vi "MoveServo_R3.vi"(6 "DIO Ref Out":T1, 8 "VISA resource name out":refnum<visa-resource-name>, 9 "GP - Low Byte":string=" ", 10 "GP - High Byte":string="\u0000", 11 "Servo ID":string="\u0001") -> (2 "Valid Checksum":bool=TRUE, 3 "Error":u64)   [LabVIEW 2015]
uses:
  <vilib>/myRIO/Instrument Drivers/Onboard IO/DIO/typedefs/DIO Reference.ctl
  <vilib>/myRIO/Common/Instrument Driver Framework/Utilities/typedefs/myRIO Generic Hardware Reference.ctl
  <vilib>/myRIO/Common/Instrument Driver Framework/Utilities/typedefs/Hardware Version Enum.ctl
  <vilib>/myRIO/Common/Instrument Driver Framework/Utilities/typedefs/myRIO v1.0 Reference.ctl
  <vilib>/myRIO/Common/Instrument Driver Framework/Utilities/typedefs/Generic FPGA Reference.ctl
  <vilib>/myRIO/Common/Instrument Driver Framework/myRIO v1.0/DIO/typedefs/DIO Channels List.ctl
  <vilib>/myRIO/Common/Instrument Driver Framework/myRIO v1.0/DIO/typedefs/DIO Channels Enum.ctl
  <vilib>/Utility/error.llb/Error Cluster From Error Code.vi
  <vilib>/myRIO/Common/Instrument Driver Framework/myRIO v1.0/DIO/vis/myRIO v1.0 Write DIO.vi
  <vilib>/myRIO/Instrument Drivers/Onboard IO/DIO/DIO.lvlib
panel:
  out "Checksum":string
  out "Tx Packet":string
  out "Calc Cksm":u8
  out "Received\nCksm":u8
  out "Received\nArray":u8[](array[numeric])
  in  "Transmit \nDelay (us)":i32=850
  in  "Return\nDelay (us)":i32=1000
  in  "RECEIVE (F)":bool[](array[boolean])=[FALSE]
  in  "TRANSMIT (T)":bool[](array[boolean])=[TRUE]
  out "Received String Array":string[](array[string])
  out "Received String":string
  # "SEND VALUES"
  # "RECEIVED VALUES"
  # "OUTPUT VALUES"
  # "INPUT"
  # "Config Parameters"
  # "Tx/Rx Delays"
  # "UART HW needs\n2-3ms to process signal\nkeeping at 2.5ms to be safe"
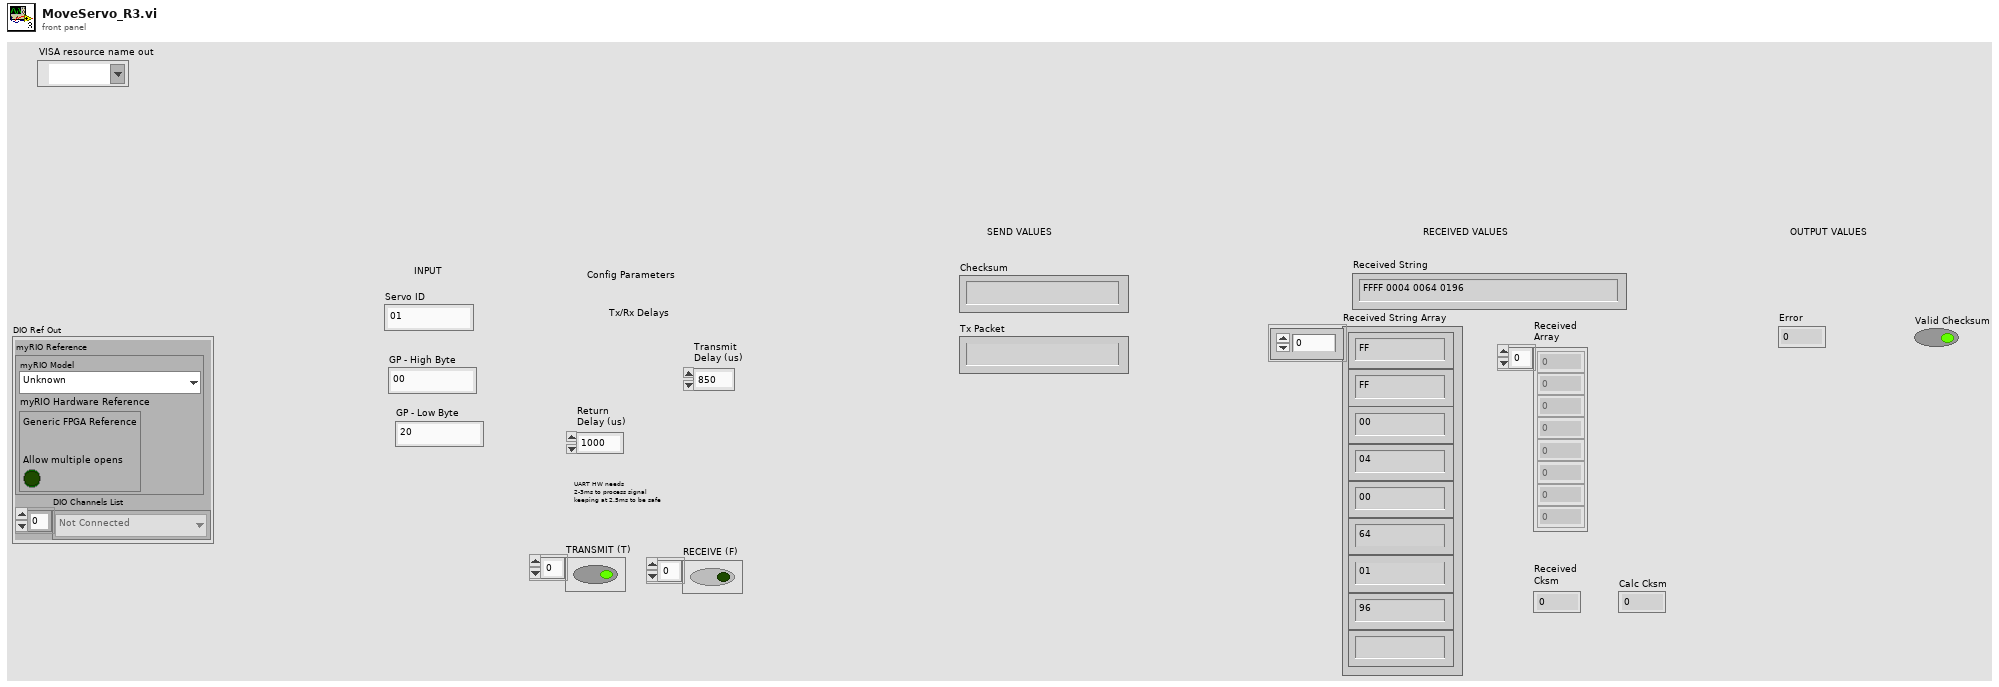
[diagram p1: front panel]
types:
  T1 = typedef "DIO.lvlib/DIO Reference.ctl" = cluster{"myRIO Reference":T2, "DIO Channels List":T6}
  T2 = typedef "myRIO Generic Hardware Reference.ctl" = cluster{"myRIO Model":T3, "myRIO Hardware Reference":T4}
  T3 = typedef "Hardware Version Enum.ctl" = enum16{"Unknown", "myRIO-1900", "myRIO-1950", "roboRIO"}
  T4 = typedef "myRIO v1.0 Reference.ctl" = cluster{"Generic FPGA Reference":T5, "Allow multiple opens":bool}
  T5 = typedef "Generic FPGA Reference.ctl" = refnum<k20>
  T6 = typedef "DIO Channels List.ctl" = T7[]
  T7 = typedef "DIO Channels Enum.ctl" = enum16{"Not Connected", "C/DIO0", "C/DIO1", "C/DIO2", "C/DIO3", "C/DIO4", "C/DIO5", "C/DIO6", "C/DIO7", "A/DIO0", "A/DIO1", "A/DIO2", "A/DIO3", "A/DIO4", "A/DIO5", "A/DIO6", "A/DIO7", "A/DIO8", "A/DIO9", "A/DIO10", "A/DIO11", "A/DIO12", "A/DIO13", "A/DIO14", "A/DIO15", "B/DIO0", "B/DIO1", "B/DIO2", "B/DIO3", "B/DIO4", "B/DIO5", "B/DIO6", "B/DIO7", "B/DIO8", "B/DIO9", "B/DIO10", "B/DIO11", "B/DIO12", "B/DIO13", "B/DIO14", "B/DIO15", "LED0", "LED1", "LED2", "LED3", "Button0", "DIO/DIO0", "DIO/DIO1", "DIO/DIO2", "DIO/DIO3", "DIO/DIO4", "DIO/DIO5", "DIO/DIO6", "DIO/DIO7", "DIO/DIO8", "DIO/DIO9", "SPI/CS0", "SPI/CS1", "SPI/CS2", "SPI/CS3", "LED RADIO (Green)", "LED RADIO (Red)", "LED COMM (Green)", "LED COMM (Red)", "LED MODE (Green)", "LED MODE (Red)"}
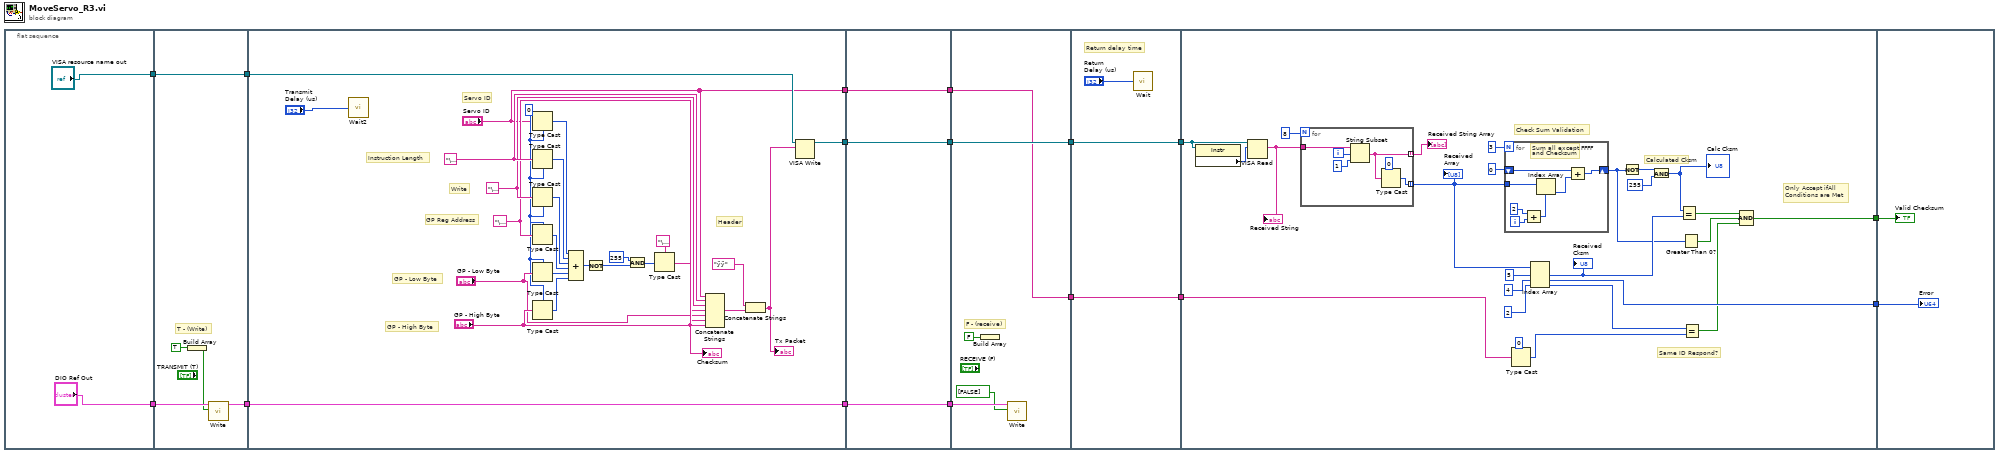
[diagram p0: block diagram]
diagram:
  n1 = flat-sequence {
    tunnel: ["VISA resource name out"] -> w16
    tunnel: ["DIO Ref Out"] -> w15
    tunnel: [w23] -> w14
    tunnel: [w20] -> w13
    tunnel: w16 -> [w20]
    tunnel: w15 -> [w21]
    tunnel: [w49] -> w12
    tunnel: [w47] -> w11
    tunnel: ["Servo ID"] -> w1
    tunnel: w13 -> [w48]
    tunnel: w14 -> [w49]
    tunnel: w12 -> [w52]
    tunnel: [w52] -> w10
    tunnel: w11 -> [w51]
    tunnel: [w51] -> w9
    tunnel: [w50] -> w2
    tunnel: w1 -> [w50]
    tunnel: w10 -> [w57]
    tunnel: w9 -> [w55]
    tunnel: [w55] -> w8
    tunnel: [w53] -> w3
    tunnel: w2 -> [w53]
    tunnel: w8 -> [w59]
    tunnel: [w59] -> w7
    tunnel: [w58] -> w4
    tunnel: w3 -> [w58]
    tunnel: w7 -> [w83]
    tunnel: [w61] -> w6
    tunnel: [w68] -> w5
    tunnel: w4 -> [w62]
    tunnel: w6 -> [w100]
    tunnel: w5 -> [w99]
    frame #0 {
    }
    frame #1 {
      # "T - (Write)"
      n2 = Build Array(TRUE) -> (w19:bool[])
      n3 = call <vilib>:"Write.vi"("Values"=w19, "DIO Ref In"=w21) -> ("DIO Ref Out"=w23:T1)  [unwired: 7 in, 1 out]
    }
    frame #2 {
      w29 = u8 0
      w34 = "\u001e"
      w35 = "\u0003"
      w36 = "\u0005"
      # "GP - High Byte"
      # "GP Reg Address"
      # "GP - Low Byte"
      # "Write"
      # "Instruction Length"
      # "Servo ID"
      # "Header"
      n4 = call "Wait2"("Count(uSec)"="Transmit \nDelay (us)") -> ()  [unwired: 1 out]
      n5 = Type Cast(type=w29, x="Servo ID") -> (*(type *) &x=w37:u8)
      n6 = Type Cast(type=w29, x=w36) -> (*(type *) &x=w38:u8)
      n7 = Type Cast(type=w29, x=w35) -> (*(type *) &x=w28:u8)
      n8 = Type Cast(type=w29, x=w34) -> (*(type *) &x=w39:u8)
      n9 = Type Cast(type=w29, x="GP - Low Byte") -> (*(type *) &x=w40:u8)
      n10 = Type Cast(type=w29, x="GP - High Byte") -> (*(type *) &x=w27:u8)
      n11 = Compound Arithmetic op=ADD(w37, w38, w28, w39, w40, w27) -> (w41:u8)
      n12 = Not(x=w41) -> (.not. x?=w43:u8)
      n13 = And(x=u8 255, y=w43) -> (x .and. y?=w45:u8)
      n14 = Type Cast(type="\u0000", x=w45) -> (*(type *) &x=w46:string)
      "Checksum" <- w46
      n15 = Concatenate Strings("Servo ID", w36, w35, w34, "GP - Low Byte", "GP - High Byte", w46) -> (w31:string)
      n16 = Concatenate Strings("ÿÿ", w31) -> (w26:string)
      "Tx Packet" <- w26
      n17 = VISA Write(VISA resource name=w48, write buffer=w26) -> (VISA resource name out=w47:refnum<visa-resource-name>)  [unwired: 1 in, 2 out]
    }
    frame #3 {
    }
    frame #4 {
      # "F - (receive)"
      n18 = Build Array(FALSE) -> ()  [unwired: 1 out]
      n19 = call <vilib>:"Write.vi"("Values"=bool[] [FALSE], "DIO Ref In"=w57) -> ()  [unwired: 7 in, 2 out]
    }
    frame #5 {
      # "Return delay time"
      n20 = call "Wait"("Count(uSec)"="Return\nDelay (us)") -> ()  [unwired: 1 out]
    }
    frame #6 {
      # "Only Accept ifAll\nConditions are Met"
      # "Same ID Respond?"
      # "Calculated Cksm"
      # "Check Sum Validation"
      n21 = property class="Instr"(reference=w83) -> ("Serial Settings:Number of Bytes at Serial Port"=w82:u32)  [unwired: 1 in, 2 out]
      n22 = VISA Read(VISA resource name=w83, byte count=w82) -> (read buffer=w84:string)  [unwired: 1 in, 3 out]
      "Received String" <- w84
      n23 = for {
        N: 8 -> [_]
        tunnel: w84 -> [w98]
        tunnel: [w94] -> w81 mode=indexing
        tunnel: [w93] -> w79 mode=indexing
        i -> [w97]
        n24 = String Subset(string=w98, offset (0)=w97, length (rest)=1) -> (substring=w94:string)
        n25 = Type Cast(type=u8 0, x=w94) -> (*(type *) &x=w93:u8)
      }
      "Received String Array" <- w81
      "Received\nArray" <- w79
      n26 = for {
        N: 3 -> [_]
        tunnel: w79 -> [w89]
        shift-right: [w88] -> w72
        shift-left: u8 0 -> [w87]
        i -> [w92]
        # "Sum all except FFFF\nand Checksum"
        n27 = Add(x=2, y=w92) -> (x+y=w90:i32)
        n28 = Index Array(array=w89, index=w90) -> (element=w86:u8)
        n29 = Add(x=w87, y=w86) -> (x+y=w88:u8)
      }
      n30 = Type Cast(type=u8 0, x=w62) -> (*(type *) &x=w63:u8)
      n31 = Index Array(array=w79, index #1=5 ("x"), index #2=4 ("x"), index #3=2 ("x")) -> (element #1=w73:u8, element #2=w68:u8, element #3=w65:u8)
      "Received\nCksm" <- w73
      n32 = Not(x=w72) -> (.not. x?=w76:u8)
      n33 = And(x=w76, y=u8 255) -> (x .and. y?=w74:u8)
      "Calc Cksm" <- w74
      n34 = Equal?(x=w74, y=w73) -> (x = y?=w71:bool)
      n35 = Greater Than 0?(x=w72) -> (x > 0?=w70:bool)
      n36 = Equal?(x=w65, y=w63) -> (x = y?=w64:bool)
      n37 = Compound Arithmetic op=AND(w71, w70, w64) -> (w61:bool)
    }
    frame #7 {
      "Valid Checksum" <- w100
      "Error" <- w99
    }
  }
